vi "SC_schleife_T_control.vi"() -> ()   [LabVIEW 2019]
uses:
  Monitors/Utility/Monitor Communication/LS370/LS370-Control.ctl
  Global/Global Variables/global.vi
  Instrument_Setup.vi
  Monitors/Utility/Monitor Communication/sub-vis/LS370_Open_Queue.vi
  Global/Global Variables/Data_Display_global.vi
  <vilib>/Analysis/NI_AALPro.lvlib
  <vilib>/Analysis/NI_AALBase.lvlib
panel:
  out "XY Graph":T1(graph)
  out "Numeric 4":dbl format="%#_13g"
  out "Numeric 5":dbl format="%#_13g"
  out "XY Graph 2":T1(graph)
  out "Array":dbl[](array[numeric])
  out "Numeric":dbl format="%#_13g"
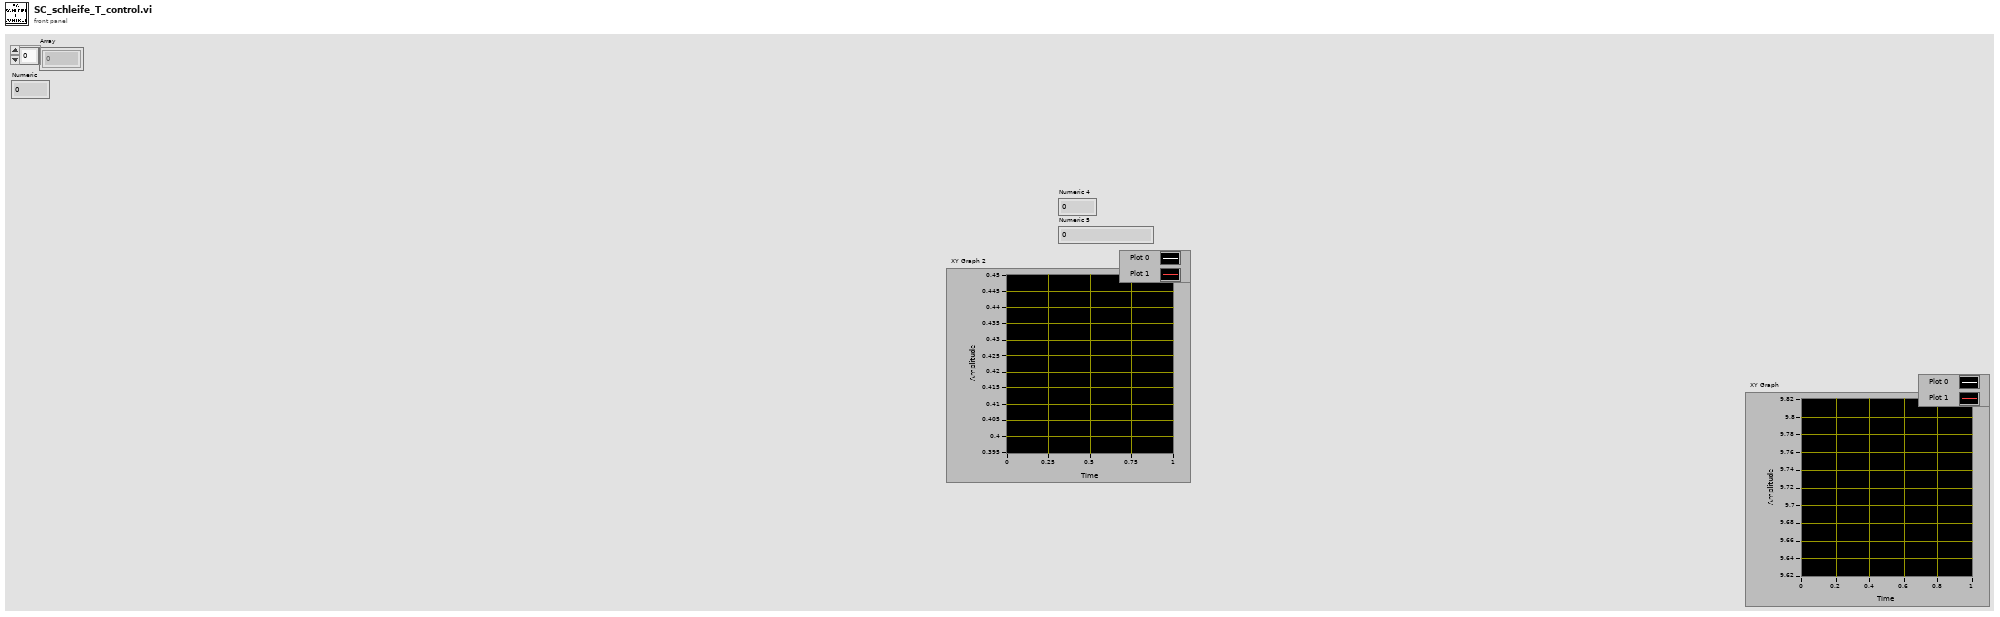
[diagram p1: front panel]
types:
  T1 = cluster{"Plot1":dbl[], "Best Linear Fit":dbl[]}[]
  T2 = typedef "LS370-Control.ctl" = cluster{"Disable Heater":bool, "Activate Tsweep":bool, "Update Lakeshores":bool, "Setpoint - Manual":dbl, "Rate (K/min)":dbl, "Sorb Power (mW)":dbl, "Still Power (mW)":dbl, "Sorb Heater":bool, "Still Heater":bool, "Set Temperature Sweep Main":bool}
  T3 = typedef "LS372-Cluster.ctl" = cluster{"Activate Tsweep":bool, "Setpoint - Manual":dbl, "Rate (K/min)":dbl, "Update Lakeshores":bool, "Still Heater":bool, "Still Power (mW)":dbl, "Manual Heater":bool, "Manual Heater  (mW) ":dbl, "Heater Range":dbl, "P (Gain)":dbl, "I (Reset)":dbl, "D (Rate)":dbl, "Heater Power (mW)":dbl, "MC Thermometer":u16, "MC Temperature":dbl, "LS372-T1":dbl, "LS372 -T2":dbl, "LS372-R1 ":dbl, "LS372-R2":dbl, "LS372-T3":dbl, "LS372-T4":dbl, "LS372-R3 ":dbl, "LS372-R4 \n\n\n\n":dbl, "LS372-T5":dbl, "LS372-T6":dbl, "LS372-R5":dbl, "LS372-R6 ":dbl, "Still Power ist":dbl, "Set Temperatur Sweep main":bool, "Setpoint ist":dbl, "Disable Heater":bool}
  T4 = typedef "Ls372-Control.ctl" = cluster{"Activate Tsweep":bool, "Setpoint - Manual":dbl, "Rate (K/min)":dbl, "Update Lakeshores":bool, "Still Heater":bool, "Still Power (mW)":dbl, "Manual Heater":bool, "Manual Heater  (mW) ":dbl, "MC Thermometer":u16, "Set Temperature Sweeep main":bool, "Disable Heater":bool}
  T5 = typedef "P9P14-TCluster.ctl" = cluster{"Setpoint":dbl, "Rate":dbl, "Chanel 1":dbl, "Approach":u16, "Set":bool, "Temperature\nStatus":i32, "Autoshutdown":bool}
  T6 = typedef "P9P14-TCluster-Control.ctl" = cluster{"Setpoint":dbl, "Rate":dbl, "Approach":u16, "Set":bool, "Autoshutdown":bool}
  T7 = typedef "ITC503Monitor-Cluster.ctl" = cluster{"Temperatur (K)":dbl, "Setpoint (K)":dbl, "Rate (K/min)":dbl, "Heater (%)":dbl, "NV (%)":dbl, "Heater Manual":bool, "NV Manual":bool, "Go to Set":bool, "Heater SP":dbl, "Valid?":bool, "Set Heater SP":bool, "Set NV SP":bool, "Heater (%) Display":dbl, "NV (%) Display":dbl, "NV Setpoint":dbl, "Change Heater Status":bool, "Change NV Status":bool, "Sample 3":dbl, "Sample 2":dbl, "Sweep-State":bool, "Set Auto PID":bool, "Auto PID":bool, "Stopp":bool, "Setpoint-Sweep":dbl, "Sample 1":dbl, "Control Channel":bool, "Channel 1":bool, "Channel 2":bool, "Channel 3":bool}
  T8 = typedef "ITC503_control.ctl" = cluster{"Setpoint (K)":dbl, "Rate (K/min)":dbl, "Go to Set":bool, "Set Heater SP":bool, "Set NV SP":bool, "Change Heater Status":bool, "Change NV Status":bool, "Set Auto PID":bool, "Stopp":bool, "Control Channel":bool, "Heater SP":dbl, "NV Setpoint":dbl}
  T9 = typedef "LS350-cluster.ctl" = cluster{"Setpoint":dbl, "Heater Output":dbl, "Setpoint control":dbl, "Enable Setpoint":bool, "LS350 T1":dbl, "LS350 T2":dbl, "LS350 T3":dbl, "LS350 T4":dbl, "LS350 R1":dbl, "LS350 R2":dbl, "LS350 R3":dbl, "LS350 R4":dbl}
  T10 = cluster{"Plot 1":dbl[], "Best Linear Fit":dbl[]}[]
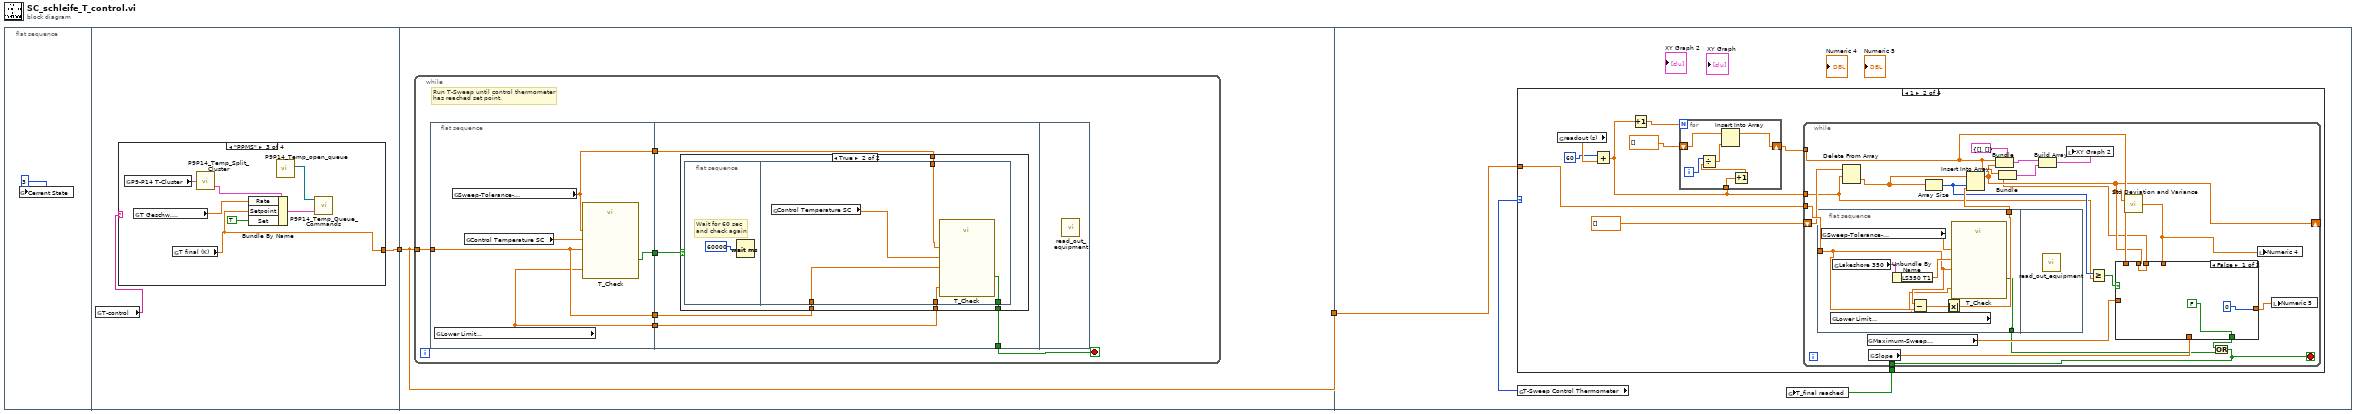
[diagram p0: block diagram]
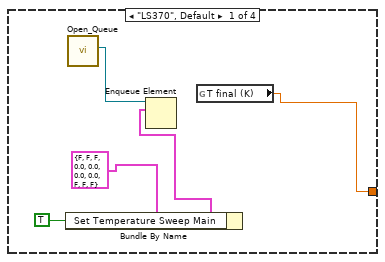
[diagram p2: hidden frame]
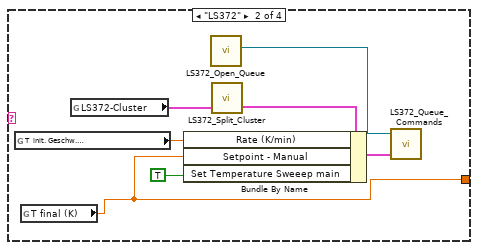
[diagram p3: hidden frame]
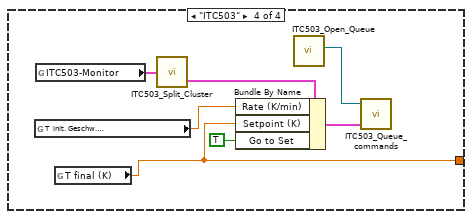
[diagram p4: hidden frame]
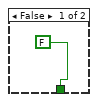
[diagram p5: hidden frame]
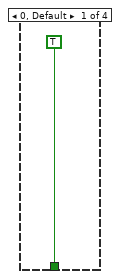
[diagram p6: hidden frame]
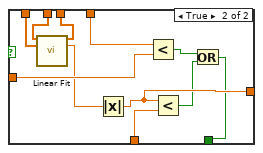
[diagram p7: hidden frame]
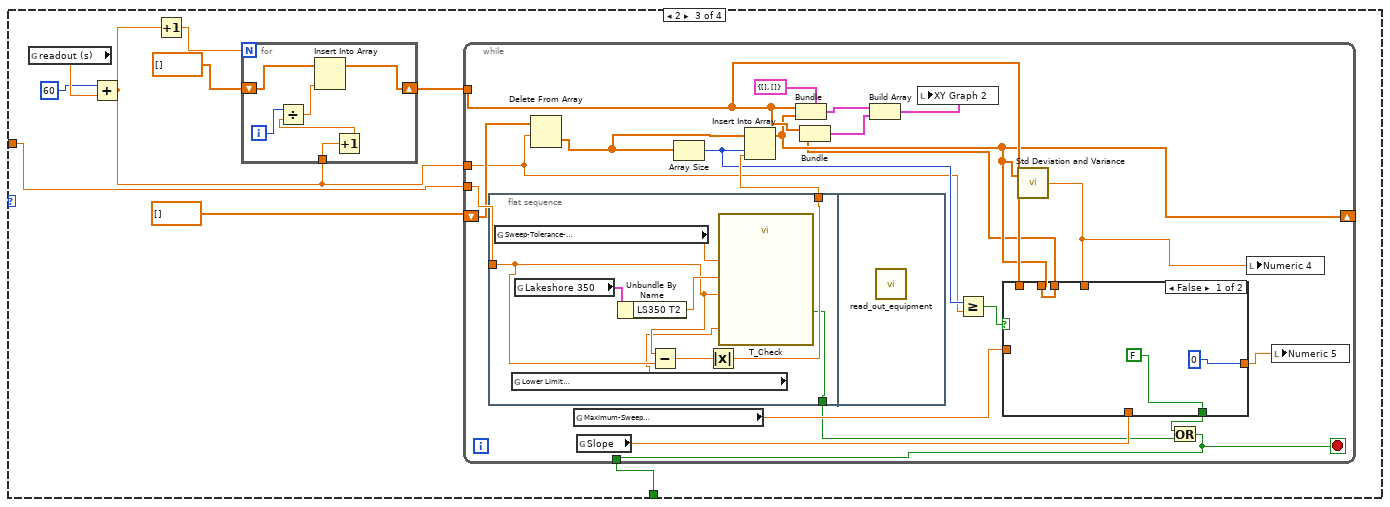
[diagram p8: hidden frame]
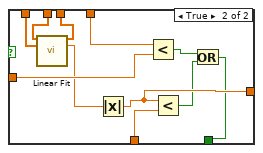
[diagram p9: hidden frame]
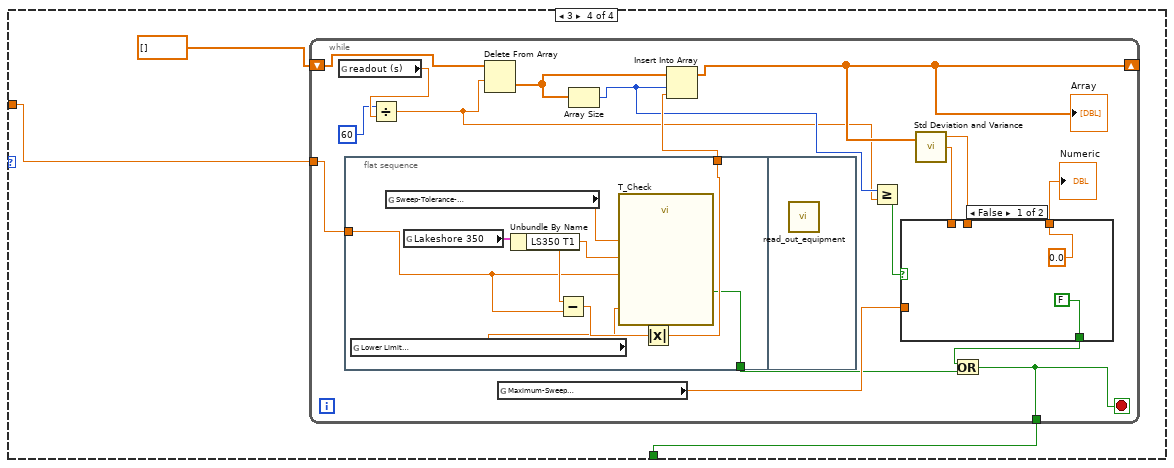
[diagram p10: hidden frame]
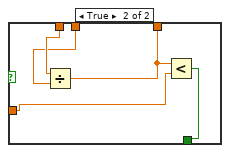
[diagram p11: hidden frame]
diagram:
  n1 = flat-sequence {
    tunnel: [w5] -> w2
    tunnel: w2 -> [w32]
    tunnel: [w32] -> w1
    tunnel: w1 -> [w61]
    frame #0 {
      n2 = global write "global.vi" "Cerrent State"(3) -> ()
    }
    frame #1 {
      n3 = global read "Instrument_Setup.vi" "T-control"() -> (w4:string)
      n4 = case shown="\"PPMS\"" w4 {
        tunnel: [w6 w11 w18 w25] -> w5
        frame "LS370", Default {
          n5 = Bundle By Name(cluster=T2 {"Disable Heater"=FALSE, "Activate Tsweep"=FALSE, "Update Lakeshores"=FALSE, "Setpoint - Manual"=0.0, "Rate (K/min)"=0.0, "Sorb Power (mW)"=0.0, "Still Power (mW)"=0.0, "Sorb Heater"=FALSE, "Still Heater"=FALSE, "Set Temperature Sweep Main"=FALSE} ("JT-Cluster"), "Set Temperature Sweep Main"=TRUE) -> (w7:T2)
          n6 = call-poly "Open_Queue.vi"() -> ("queue out"=w10:refnum<queue>)  [unwired: 10 in, 1 out]
          n7 = Enqueue Element(queue=w10, element=w7) -> ()  [unwired: 2 in, 3 out]
          n8 = global read "global.vi" "T final (K)"() -> (w6:dbl)
        }
        frame "LS372" {
          n9 = global read "global.vi" "T  init. Geschw. \n(K/min)"() -> (w14:dbl)
          n10 = global read "global.vi" "T final (K)"() -> (w11:dbl)
          n11 = global read "Data_Display_global.vi" "LS372-Cluster"() -> (w17:T3)
          n12 = call "LS372_Open_Queue.vi"() -> ("queue out"=w13:refnum<queue>)  [unwired: 10 in, 1 out]
          n13 = call "LS372_Split_Cluster.vi"("LS372-Cluster"=w17) -> ("LS372-Control"=w16:T4)  [unwired: 1 out]
          n14 = Bundle By Name(cluster=w16, "Rate (K/min)"=w14, "Setpoint - Manual"=w11, "Set Temperature Sweeep main"=TRUE) -> (w12:T4)
          n15 = call "LS372_Queue_Commands.vi"("LS372-Control"=w12, "Queue"=w13) -> ()  [unwired: 1 in, 1 out]
        }
        frame "PPMS" {
          n16 = global read "Data_Display_global.vi" "P9-P14 T-Cluster"() -> (w19:T5)
          n17 = global read "global.vi" "T Geschw. \n(K/min)"() -> (w24:dbl)
          n18 = global read "global.vi" "T final (K)"() -> (w18:dbl)
          n19 = call "P9P14_Temp_Split_Cluster.vi"("P9-P14 T-Cluster"=w19) -> ("P9-P14 T-Cluster -Control"=w20:T6)  [unwired: 1 out]
          n20 = Bundle By Name(cluster=w20, "Rate"=w24, "Setpoint"=w18, "Set"=TRUE) -> (w22:T6)
          n21 = call "P9P14_Temp_open_queue.vi"() -> ("queue out"=w23:refnum<queue>)  [unwired: 10 in, 1 out]
          n22 = call "P9P14_Temp_Queue_Commands.vi"("P9-P14 T-Cluster -Control"=w22, "Queue"=w23) -> ()  [unwired: 1 in, 1 out]
        }
        frame "ITC503" {
          n23 = global read "global.vi" "T  init. Geschw. \n(K/min)"() -> (w31:dbl)
          n24 = global read "Data_Display_global.vi" "ITC503-Monitor"() -> (w29:T7)
          n25 = global read "global.vi" "T final (K)"() -> (w25:dbl)
          n26 = call "ITC503_Split_Cluster.vi"("ITC503-Monitor"=w29) -> ("ITC503-Control"=w28:T8)  [unwired: 1 out]
          n27 = Bundle By Name(cluster=w28, "Rate (K/min)"=w31, "Setpoint (K)"=w25, "Go to Set"=TRUE) -> (w27:T8)
          n28 = call "ITC503_Open_Queue.vi"() -> ("queue out"=w30:refnum<queue>)  [unwired: 10 in, 1 out]
          n29 = call "ITC503_Queue_commands.vi"("ITC503-Control"=w27, "ITC503 Queue"=w30) -> ()  [unwired: 1 in, 1 out]
        }
      }
    }
    frame #2 {
      n30 = while {
        tunnel: w32 -> [w38]
        stop <- w34 stop-if-true
        # "Run T-Sweep until control thermometer\nhas reached set point."
        n31 = flat-sequence {
          tunnel: w38 -> [w41]
          tunnel: [w42] -> w37
          tunnel: [w41] -> w36
          tunnel: [w40] -> w35
          tunnel: [w39] -> w33
          tunnel: w37 -> [w48]
          tunnel: w36 -> [w47]
          tunnel: w35 -> [w46]
          tunnel: [w45] -> w34
          tunnel: w33 -> [w44]
          frame #0 {
            n32 = global read "Instrument_Setup.vi" "Lower Limit\nSweep-Tolerance-\nTemperature (K)"() -> (w39:dbl)
            n33 = global read "Instrument_Setup.vi" "Sweep-Tolerance-\nTemperature (%)"() -> (w42:dbl)
            n34 = global read "Data_Display_global.vi" "Control Temperature SC"() -> (w43:dbl)
            n35 = call "T_Check.vi"("Lower Limit Sweep\nTolerance (K)"=w39, "T_target (K)"=w41, "Sweep\nTolerance %"=w42, "T_in"=w43) -> ("= T target"=w40:bool)
          }
          frame #1 {
            n36 = case shown="True" w46 {
              tunnel: w47 -> [_ w53]
              tunnel: w48 -> [_ w52]
              tunnel: [FALSE w51] -> w45
              tunnel: w44 -> [_ w50]
              frame False {
              }
              frame True {
                n37 = flat-sequence {
                  tunnel: w53 -> [w59]
                  tunnel: w52 -> [w58]
                  tunnel: [w57] -> w51
                  tunnel: w50 -> [w55]
                  frame #0 {
                    # "Wait for 60 sec\nand check again"
                    n38 = Wait (ms)(milliseconds to wait=60000) -> ()  [unwired: 1 out]
                  }
                  frame #1 {
                    n39 = global read "Data_Display_global.vi" "Control Temperature SC"() -> (w56:dbl)
                    n40 = call "T_Check.vi"("Lower Limit Sweep\nTolerance (K)"=w55, "T_target (K)"=w59, "Sweep\nTolerance %"=w58, "T_in"=w56) -> ("= T target"=w57:bool)
                  }
                }
              }
            }
          }
          frame #2 {
            n41 = call "read_out_equipment.vi"() -> ()  [unwired: 1 in]
          }
        }
      }
    }
    frame #3 {
      n42 = global read "Instrument_Setup.vi" "T-Sweep Control Thermometer"() -> (w62:u16)
      n43 = case shown="1" w62 {
        tunnel: w61 -> [_ w67 w123 w182]
        tunnel: [TRUE w64 w130 w180] -> w60
        frame 0, Default {
        }
        frame 1 {
          n44 = global read "Instrument_Setup.vi" "readout (s)"() -> (w72:dbl)
          n45 = Add(x=60, y=w72) -> (x+y=w65:dbl)
          n46 = Increment(x=w65) -> (x+1=w70:dbl)
          n47 = for {
            N: w70 -> [_]
            shift-right: [w118] -> w66
            shift-left: dbl[] [] -> [w120]
            tunnel: w65 -> [w117]
            i -> [w121]
            n48 = Increment(x=w117) -> (x+1=w116:dbl)
            n49 = Divide(x=w121, y=w116) -> (x/y=w119:dbl)
            n50 = Insert Into Array(array=w120, new element=w119) -> (w118:dbl[])  [unwired: 1 in]
          }
          n51 = while {
            shift-right: [w82] -> _
            shift-left: dbl[] [] -> [w92]
            tunnel: w67 -> [w93]
            tunnel: w66 -> [w85]
            tunnel: w65 -> [w83]
            tunnel: [w73] -> w64
            stop <- w73 stop-if-true
            n52 = flat-sequence {
              tunnel: w93 -> [w112]
              tunnel: [w110] -> w89
              tunnel: [w109] -> w75
              frame #0 {
                n53 = global read "Instrument_Setup.vi" "Sweep-Tolerance-\nTemperature (%)"() -> (w115:dbl)
                n54 = global read "Instrument_Setup.vi" "Lower Limit\nSweep-Tolerance-\nTemperature (K)"() -> (w108:dbl)
                n55 = global read "Data_Display_global.vi" "Lakeshore 350"() -> (w114:T9)
                n56 = Unbundle By Name(w114) -> ("LS350 T1"=w113:dbl)
                n57 = Subtract(x=w112, y=w112) -> (x-y=w111:dbl)
                n58 = Absolute Value(x=w111) -> (abs(x)=w110:dbl)
                n59 = call "T_Check.vi"("Lower Limit Sweep\nTolerance (K)"=w108, "T_target (K)"=w112, "Sweep\nTolerance %"=w115, "T_in"=w113) -> ("= T target"=w109:bool)
              }
              frame #1 {
                n60 = call "read_out_equipment.vi"() -> ()  [unwired: 1 in]
              }
            }
            n61 = Delete From Array(array=w92, length=w83) -> (deleted portion=w90:dbl[])  [unwired: 1 in, 1 out]
            n62 = global read "Instrument_Setup.vi" "Maximum-Sweep\nSettle %/min"() -> (w78:dbl)
            n63 = global read "Instrument_Setup.vi" "Slope"() -> (w77:dbl)
            n64 = Array Size(array=w90) -> (size(s)=w84:i32)
            n65 = Insert Into Array(array=w90, index=w84, new element=w89) -> (w82:dbl[])
            n66 = Bundle(cluster=cluster{"Plot 1":dbl[], "Plot 2":dbl[]} {"Plot 1"=[], "Plot 2"=[]}, "Plot 1"=w85, "Plot 2"=w82) -> (w88:cluster{"Plot 1":dbl[], "Plot 2":dbl[]})
            n67 = Greater Or Equal?(x=w84, y=w83) -> (x >= y?=w79:bool)
            n68 = call <vilib>:"Std Deviation and Variance.vi"("X"=w82) -> ("standard deviation"=w81:dbl)  [unwired: 1 in, 2 out]
            n69 = case shown="False" w79 {
              tunnel: w82 -> [w94 w106]
              tunnel: w85 -> [_ w107]
              tunnel: w81 -> [_ w104]
              tunnel: [w94 w105] -> w80
              tunnel: w78 -> [_ w103]
              tunnel: w77 -> [_ w101]
              tunnel: [0 w100] -> w76
              tunnel: [FALSE w97] -> w74
              frame False {
              }
              frame True {
                n70 = call <vilib>:"Linear Fit.vi"("Y"=w106, "X"=w107) -> ("Best Linear Fit"=w105:dbl[], "slope"=w102:dbl)  [unwired: 9 in, 3 out]
                n71 = Absolute Value(x=w102) -> (abs(x)=w100:dbl)
                n72 = Less?(x=w104, y=w103) -> (x < y?=w99:bool)
                n73 = Less?(x=w100, y=w101) -> (x < y?=w98:bool)
                n74 = Or(x=w99, y=w98) -> (x .or. y?=w97:bool)
              }
            }
            n75 = Bundle(w85, "Best Linear Fit"=w80) -> (w87:cluster{dbl[], "Best Linear Fit":dbl[]})  [unwired: 1 in]
            n76 = Build Array(w88, w87) -> (w86:T10)
            n77 = local write "XY Graph 2"(w86) -> ()
            n78 = Or(x=w74, y=w75) -> (x .or. y?=w73:bool)
            n79 = local write "Numeric 4"(w81) -> ()
            n80 = local write "Numeric 5"(w76) -> ()
          }
        }
        frame 2 {
          n81 = global read "Instrument_Setup.vi" "readout (s)"() -> (w129:dbl)
          n82 = Add(x=60, y=w129) -> (x+y=w124:dbl)
          n83 = Increment(x=w124) -> (x+1=w127:dbl)
          n84 = for {
            N: w127 -> [_]
            shift-right: [w133] -> w125
            shift-left: dbl[] [] -> [w135]
            tunnel: w124 -> [w132]
            i -> [w136]
            n85 = Increment(x=w132) -> (x+1=w131:dbl)
            n86 = Divide(x=w136, y=w131) -> (x/y=w134:dbl)
            n87 = Insert Into Array(array=w135, new element=w134) -> (w133:dbl[])  [unwired: 1 in]
          }
          n88 = while {
            shift-right: [w146] -> _
            shift-left: dbl[] [] -> [w156]
            tunnel: w123 -> [w157]
            tunnel: w125 -> [w149]
            tunnel: w124 -> [w147]
            tunnel: [w137] -> w130
            stop <- w137 stop-if-true
            n89 = flat-sequence {
              tunnel: w157 -> [w176]
              tunnel: [w174] -> w153
              tunnel: [w173] -> w139
              frame #0 {
                n90 = global read "Instrument_Setup.vi" "Sweep-Tolerance-\nTemperature (%)"() -> (w179:dbl)
                n91 = global read "Instrument_Setup.vi" "Lower Limit\nSweep-Tolerance-\nTemperature (K)"() -> (w172:dbl)
                n92 = global read "Data_Display_global.vi" "Lakeshore 350"() -> (w178:T9)
                n93 = Unbundle By Name(w178) -> ("LS350 T2"=w177:dbl)
                n94 = Subtract(x=w176, y=w176) -> (x-y=w175:dbl)
                n95 = Absolute Value(x=w175) -> (abs(x)=w174:dbl)
                n96 = call "T_Check.vi"("Lower Limit Sweep\nTolerance (K)"=w172, "T_target (K)"=w176, "Sweep\nTolerance %"=w179, "T_in"=w177) -> ("= T target"=w173:bool)
              }
              frame #1 {
                n97 = call "read_out_equipment.vi"() -> ()  [unwired: 1 in]
              }
            }
            n98 = Delete From Array(array=w156, length=w147) -> (deleted portion=w154:dbl[])  [unwired: 1 in, 1 out]
            n99 = global read "Instrument_Setup.vi" "Maximum-Sweep\nSettle %/min"() -> (w142:dbl)
            n100 = global read "Instrument_Setup.vi" "Slope"() -> (w141:dbl)
            n101 = Array Size(array=w154) -> (size(s)=w148:i32)
            n102 = Insert Into Array(array=w154, index=w148, new element=w153) -> (w146:dbl[])
            n103 = Bundle(cluster=cluster{"Plot 1":dbl[], "Plot 2":dbl[]} {"Plot 1"=[], "Plot 2"=[]}, "Plot 1"=w149, "Plot 2"=w146) -> (w152:cluster{"Plot 1":dbl[], "Plot 2":dbl[]})
            n104 = Greater Or Equal?(x=w148, y=w147) -> (x >= y?=w143:bool)
            n105 = call <vilib>:"Std Deviation and Variance.vi"("X"=w146) -> ("standard deviation"=w145:dbl)  [unwired: 1 in, 2 out]
            n106 = case shown="False" w143 {
              tunnel: w146 -> [w158 w170]
              tunnel: w149 -> [_ w171]
              tunnel: w145 -> [_ w168]
              tunnel: [w158 w169] -> w144
              tunnel: w142 -> [_ w167]
              tunnel: w141 -> [_ w165]
              tunnel: [0 w164] -> w140
              tunnel: [FALSE w161] -> w138
              frame False {
              }
              frame True {
                n107 = call <vilib>:"Linear Fit.vi"("Y"=w170, "X"=w171) -> ("Best Linear Fit"=w169:dbl[], "slope"=w166:dbl)  [unwired: 9 in, 3 out]
                n108 = Absolute Value(x=w166) -> (abs(x)=w164:dbl)
                n109 = Less?(x=w168, y=w167) -> (x < y?=w163:bool)
                n110 = Less?(x=w164, y=w165) -> (x < y?=w162:bool)
                n111 = Or(x=w163, y=w162) -> (x .or. y?=w161:bool)
              }
            }
            n112 = Bundle(w149, "Best Linear Fit"=w144) -> (w151:cluster{dbl[], "Best Linear Fit":dbl[]})  [unwired: 1 in]
            n113 = Build Array(w152, w151) -> (w150:T10)
            n114 = local write "XY Graph 2"(w150) -> ()
            n115 = Or(x=w138, y=w139) -> (x .or. y?=w137:bool)
            n116 = local write "Numeric 4"(w145) -> ()
            n117 = local write "Numeric 5"(w140) -> ()
          }
        }
        frame 3 {
          n118 = while {
            tunnel: w182 -> [w195]
            shift-right: [w193] -> _
            shift-left: dbl[] [] -> [w197]
            tunnel: [w183] -> w180
            stop <- w183 stop-if-true
            n119 = global read "Instrument_Setup.vi" "readout (s)"() -> (w199:dbl)
            n120 = flat-sequence {
              tunnel: w195 -> [w211]
              tunnel: [w209] -> w194
              tunnel: [w208] -> w184
              frame #0 {
                n121 = global read "Instrument_Setup.vi" "Lower Limit\nSweep-Tolerance-\nTemperature (K)"() -> (w207:dbl)
                n122 = global read "Instrument_Setup.vi" "Sweep-Tolerance-\nTemperature (%)"() -> (w214:dbl)
                n123 = global read "Data_Display_global.vi" "Lakeshore 350"() -> (w213:T9)
                n124 = Unbundle By Name(w213) -> ("LS350 T1"=w212:dbl)
                n125 = Subtract(x=w212, y=w211) -> (x-y=w210:dbl)
                n126 = call "T_Check.vi"("Lower Limit Sweep\nTolerance (K)"=w207, "T_target (K)"=w211, "Sweep\nTolerance %"=w214, "T_in"=w212) -> ("= T target"=w208:bool)
                n127 = Absolute Value(x=w210) -> (abs(x)=w209:dbl)
              }
              frame #1 {
                n128 = call "read_out_equipment.vi"() -> ()  [unwired: 1 in]
              }
            }
            n129 = Divide(x=60, y=w199) -> (x/y=w188:dbl)
            n130 = Delete From Array(array=w197, length=w188) -> (deleted portion=w196:dbl[])  [unwired: 1 in, 1 out]
            n131 = global read "Instrument_Setup.vi" "Maximum-Sweep\nSettle %/min"() -> (w186:dbl)
            n132 = Array Size(array=w196) -> (size(s)=w189:i32)
            n133 = Insert Into Array(array=w196, index=w189, new element=w194) -> (w193:dbl[])
            "Array" <- w193
            n134 = Greater Or Equal?(x=w189, y=w188) -> (x >= y?=w187:bool)
            n135 = call <vilib>:"Std Deviation and Variance.vi"("X"=w193) -> ("mean"=w192:dbl, "standard deviation"=w191:dbl)  [unwired: 1 in, 1 out]
            n136 = case shown="False" w187 {
              tunnel: w192 -> [_ w205]
              tunnel: w191 -> [_ w206]
              tunnel: [0.0 w204] -> w190
              tunnel: w186 -> [_ w203]
              tunnel: [FALSE w202] -> w185
              frame False {
              }
              frame True {
                n137 = Divide(x=w206, y=w205) -> (x/y=w204:dbl)
                n138 = Less?(x=w204, y=w203) -> (x < y?=w202:bool)
              }
            }
            "Numeric" <- w190
            n139 = Or(x=w185, y=w184) -> (x .or. y?=w183:bool)
          }
        }
      }
      n140 = global write "Data_Display_global.vi" "T_final reached"(w60) -> ()
    }
  }
